vi "06a-arrays.vi"() -> ()   [LabVIEW 2018, in "LV-0mq-Julia_roundtrip-lib.lvlib"]
uses:
  LV-0mq-Julia_roundtrip-lib.lvlib
  Server or client state.ctl
  detailed error info.ctl
  StackFrame.ctl
  Commands.ctl
  72a46192-383e-4ee5-9465-71670922b82a.vi
  ef5408d4-6538-41d1-b296-fda05a71e4b0.vi
  d2cb43a9-9305-42fb-ad58-bce983510195.vi
  e4efb182-1b04-4d49-96a3-1defebd055ea.vi
  ebebf057-8b7e-42d1-8726-0ed76f361650.vi
  72a46192-383e-4ee5-9465-71670922b82a.vi/ea2ca31c-a649-493c-8d06-3a8000b732b1.vi
  ef5408d4-6538-41d1-b296-fda05a71e4b0.vi/365813fc-9c19-4b31-a490-477dd90e6dd4.vi
  d2cb43a9-9305-42fb-ad58-bce983510195.vi/e28c4e1c-617d-4a26-8291-f58a5accd33d.vi
  d2cb43a9-9305-42fb-ad58-bce983510195.vi/697b26af-9cff-4296-98ec-fa9d12ca8fdc.vi
  d2cb43a9-9305-42fb-ad58-bce983510195.vi/17159f77-75f5-4b7b-8d47-844af2eb1bcd.vi
  e4efb182-1b04-4d49-96a3-1defebd055ea.vi/c831fe72-f3ce-4847-96da-e1889b23ddae.vi
  e4efb182-1b04-4d49-96a3-1defebd055ea.vi/ef51326b-c369-4f95-bb54-a6ec3719e99a.vi
  ebebf057-8b7e-42d1-8726-0ed76f361650.vi/2896c3ac-7382-471b-957d-23d54ee9f1a8.vi
  ebebf057-8b7e-42d1-8726-0ed76f361650.vi/710b0f88-80e8-4b85-a109-d5d9dfaa7844.vi
  72a46192-383e-4ee5-9465-71670922b82a.vi/ea2ca31c-a649-493c-8d06-3a8000b732b1.vi/4cda02a8-52b1-4797-9517-7736628fdc16.vi
  ef5408d4-6538-41d1-b296-fda05a71e4b0.vi/365813fc-9c19-4b31-a490-477dd90e6dd4.vi/c1bf83d8-4e50-4008-8373-782bae7d23a9.vi
  e4efb182-1b04-4d49-96a3-1defebd055ea.vi/c831fe72-f3ce-4847-96da-e1889b23ddae.vi/9c4cdaea-65f9-4c6c-8a66-2fd1ac6f4f5c.vi
  e4efb182-1b04-4d49-96a3-1defebd055ea.vi/c831fe72-f3ce-4847-96da-e1889b23ddae.vi/3acea7b0-1723-4660-a8ee-e10d34bc4f15.vi
  ebebf057-8b7e-42d1-8726-0ed76f361650.vi/2896c3ac-7382-471b-957d-23d54ee9f1a8.vi/1bedb906-9d55-4714-9acf-3a7596d20d1c.vi
  ebebf057-8b7e-42d1-8726-0ed76f361650.vi/2896c3ac-7382-471b-957d-23d54ee9f1a8.vi/27a3c6cf-df38-46c5-966e-0597bcc583ab.vi
  72a46192-383e-4ee5-9465-71670922b82a.vi/ea2ca31c-a649-493c-8d06-3a8000b732b1.vi/4cda02a8-52b1-4797-9517-7736628fdc16.vi/f6bd3a2a-1504-4020-af9c-daf7937f7973.vi
  ef5408d4-6538-41d1-b296-fda05a71e4b0.vi/365813fc-9c19-4b31-a490-477dd90e6dd4.vi/c1bf83d8-4e50-4008-8373-782bae7d23a9.vi/fa26639b-d519-4ace-9d6a-dd3a988d1d0b.vi
  e4efb182-1b04-4d49-96a3-1defebd055ea.vi/c831fe72-f3ce-4847-96da-e1889b23ddae.vi/9c4cdaea-65f9-4c6c-8a66-2fd1ac6f4f5c.vi/fa7cffbf-0952-4399-bf7e-4cf3444aec21.vi
  ebebf057-8b7e-42d1-8726-0ed76f361650.vi/2896c3ac-7382-471b-957d-23d54ee9f1a8.vi/1bedb906-9d55-4714-9acf-3a7596d20d1c.vi/32202c8e-48ac-4eff-9f06-aea6b9e0f0c2.vi
  jl-scripts path.vi
  check ID validity.vi
  bindata_descr to JSON.vi
  check cluster field names.vi
  concat JSON.vi
  <vilib>/Utility/error.llb/Error Cluster From Error Code.vi
panel:
  out "inverted matrix":dbl[][](array[numeric])=[[1.0, 0.0, 5.0], [4.0, 2.0, 1.0], [2.0, 2.0, 3.0]] format="%#.4g"
  out "determinant":dbl
  out "Solution Vector":dbl[](array[numeric]) format="%.2f"
  in  "Known Vector":dbl[](array[numeric])=[22.0, 14.0, 18.0]
  in  "Input Matrix":dbl[][](array[numeric])=[[1.0, 0.0, 5.0], [4.0, 2.0, 1.0], [2.0, 2.0, 3.0]]
  in  "next":bool
  out "detailed error info":T1
  out "current error":errorcluster
  out "final error":errorcluster
  out "short err code":u8
  in  "stop":bool
  out "ZMQ timeout":bool
  out "Julia script file path":path
  out "temporary script path":path
  out "Jl Server state":T3
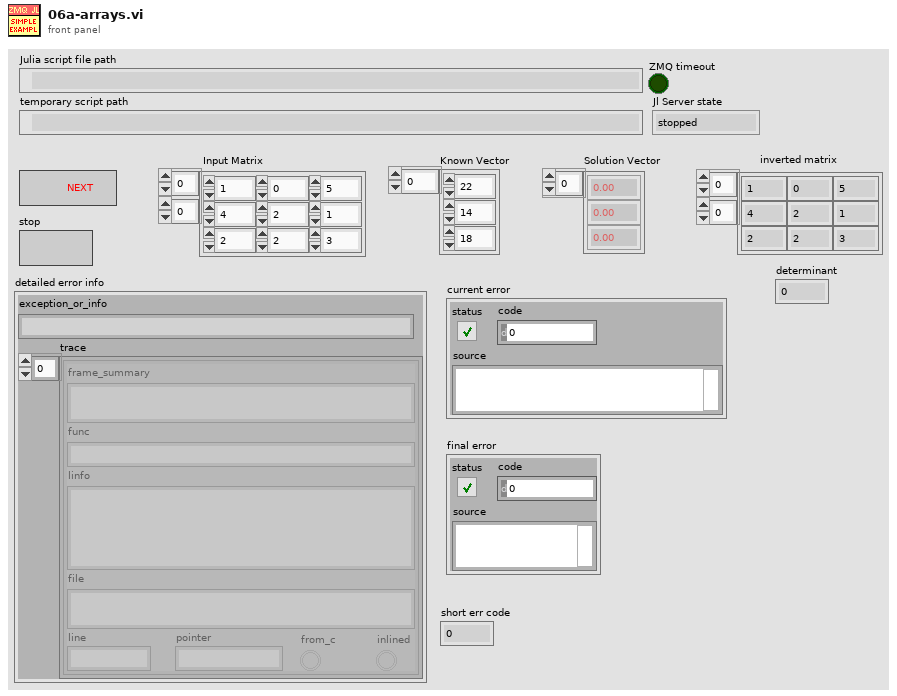
[diagram p1: front panel]
types:
  T1 = typedef "LV-0mq-Julia_roundtrip-lib.lvlib/detailed error info.ctl" = cluster{"exception_or_info":string, "trace":T2[]}
  T2 = typedef "LV-0mq-Julia_roundtrip-lib.lvlib/StackFrame.ctl" = cluster{"frame_summary":string, "func":string, "linfo":string, "file":string, "line":i32, "pointer":u64, "from_c":bool, "inlined":bool}
  T3 = typedef "LV-0mq-Julia_roundtrip-lib.lvlib/Server or client state.ctl" = enum16{"stopped", "running", "unknown"}
  T4 = typedef "LV-0mq-Julia_roundtrip-lib.lvlib/Commands.ctl" = enum16{"Start Jl-server & Init LV-client", "Send request & Get response ", "Stop Jl-server & Cleanup LV-client", "Cleanup LV-client", "Start Jl-server", "Stop Jl-server", "Init LV-Client", "Cleanup LV-Client", "(not allowed)", "Set LV Client state", "Set Jl Server state", "set ZMQ timeout", "read ZMQ timeout", "read-out state"}
  T5 = typedef "LV-0mq-Julia_roundtrip-lib.lvlib/Bindata&description.ctl" = cluster{"bindata_descr":T6[], "bindata":u8[]}
  T6 = typedef "LV-0mq-Julia_roundtrip-lib.lvlib/Bindata description.ctl" = cluster{"nofbytes":i32, "numtype":string, "start":i32, "arrdims":i32[], "kwarg_name":string, "category":string}
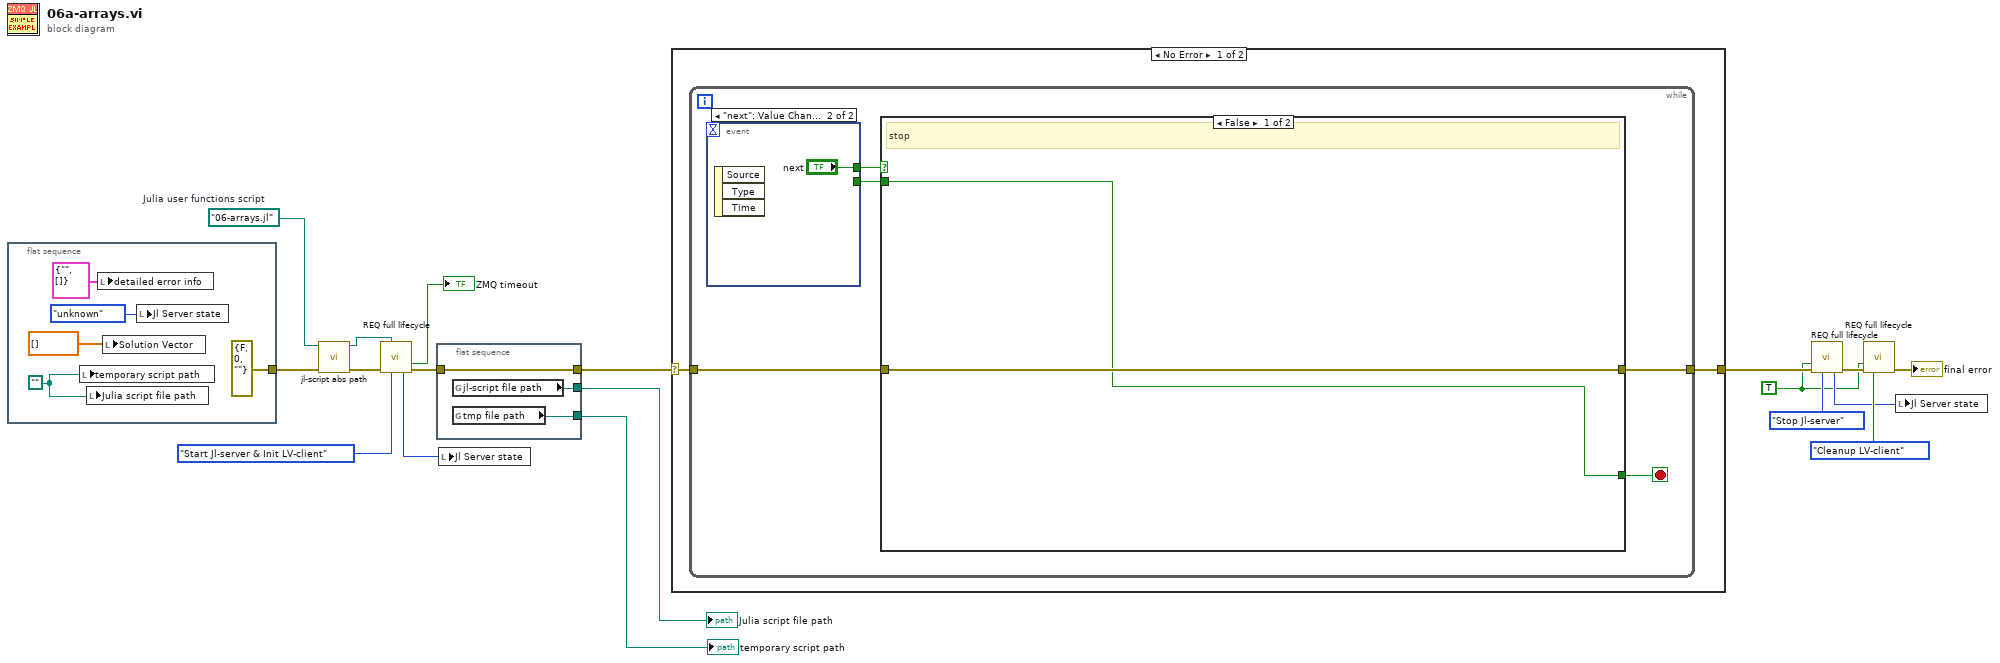
[diagram p0: block diagram]
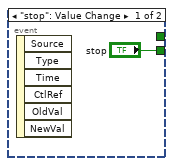
[diagram p2: hidden frame]
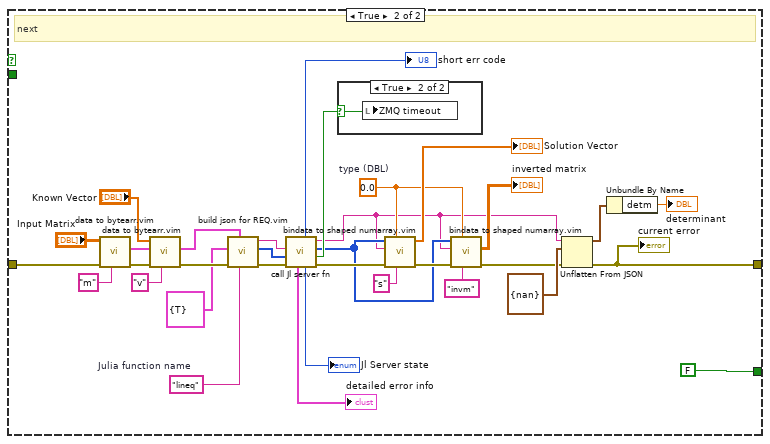
[diagram p3: hidden frame]
diagram:
  w4 = path "06-arrays.jl"  # Julia user functions script
  w1 = TRUE ("Force command")
  n1 = flat-sequence {
    tunnel: [errorcluster {"status"=FALSE, "code"=0, "source"=""} ("error in (no error)")] -> w2
    frame #0 {
      w19 = path ""
      n2 = local write "temporary script path"(w19) -> ()
      n3 = local write "Julia script file path"(w19) -> ()
      n4 = local write "detailed error info"(T1 {"exception_or_info"="", "trace"=[]} ("detailed error info")) -> ()
      n5 = local write "Solution Vector"(dbl[] [] ("Server response")) -> ()
      n6 = local write "Jl Server state"(Server_or_client_state."unknown" ("Jl Server state out")) -> ()
    }
  }
  n7 = call "jl-script abs path.vi"("error in (no error)"=w2, "Julia user functions script"=w4) -> ("error out"=w5:errorcluster, "script abs path"=w6:path)  [unwired: 8 in]
  n8 = call "REQ full lifecycle.vi"("Julia user functions script"=w6, "error in"=w5, "command"=Commands."Start Jl-server & Init LV-client") -> ("timeout?"=→"ZMQ timeout":bool, "Jl Server state out"=w8:T3, "error out"=w7:errorcluster)  [unwired: 6 in, 4 out]
  n9 = flat-sequence {
    tunnel: [w26] -> w13
    tunnel: w7 -> [w26]
    tunnel: [w25] -> w11
    tunnel: [w24] -> w12
    frame #0 {
      n10 = global read "jl-scripts path.vi" "jl-script file path"() -> (w25:path)
      n11 = global read "jl-scripts path.vi" "tmp file path"() -> (w24:path)
    }
  }
  n12 = local write "Jl Server state"(w8) -> ()
  n13 = case shown="No Error" w13 {
    selector: w13 -> [w27 w72]
    tunnel: [w28 w72] -> w18
    frame No Error {
      n14 = while {
        tunnel: w27 -> [w32]
        tunnel: [w33] -> w28
        stop <- w30 stop-if-true
        n15 = event shown="[1] \"next\": Value Change" {
          selector: _ -> [_ _]
          dyn-events: _ -> [_ _]
          timeout: _ -> [_ _]
          tunnel: [_ "next"] -> w31
          tunnel: ["stop" _] -> w29
          event "stop": Value Change {
            n16 = event-data() -> ()  [unwired: 1 in, 6 out]
          }
          event "next": Value Change {
            n17 = event-data() -> ()  [unwired: 1 in, 3 out]
          }
        }
        n18 = case shown="False" w31 {
          tunnel: [w37 w46] -> w33
          tunnel: w32 -> [w37 w56]
          tunnel: [w36 FALSE ("stop this VI only")] -> w30
          tunnel: w29 -> [w36 _]
          frame False {
            # "stop"
          }
          frame True {
            w40 = 0.0  # type (DBL)
            w62 = "lineq"  # Julia function name
            # "next"
            n19 = call "data to bytearr.vim"("kwarg_name"="m", "error in (no error)"=w56, "data in"="Input Matrix") -> ("error out"=w60:errorcluster, "Bindata & descr out"=w59:T5)  [unwired: 6 in, 1 out]
            n20 = call "data to bytearr.vim"("kwarg_name"="v", "error in (no error)"=w60, "Bindata & descr in"=w59, "data in"="Known Vector") -> ("error out"=w57:errorcluster, "Bindata & descr out"=w53:T5)  [unwired: 5 in, 1 out]
            n21 = call "build json for REQ.vim"("fun2call"=w62, "Bindata & descr in"=w53, "error in (no error)"=w57, "Arguments 2"=cluster{"invert":bool} {"invert"=TRUE}) -> ("error out"=w67:errorcluster, "bindata out"=w68:u8[], "JSON string out"=w69:string)  [unwired: 5 in]
            n22 = call "call Jl server fn.vi"("error in (no error)"=w67, "binary data in"=w68, "JSON string in"=w69) -> ("error out"=w52:errorcluster, "timeout?"=w63:bool, "binary data received"=w42:u8[], "JSON received"=w38:string, "Jl Server state out"=→"Jl Server state":T3, "return code"=→"short err code":u8, "detailed error info"=→"detailed error info":T1)  [unwired: 2 in]
            n23 = case shown="True" w63 {
              selector: w63 -> [_ w71]
              frame False {
              }
              frame True {
                n24 = local write "ZMQ timeout"(w71) -> ()
              }
            }
            n25 = call "bindata to shaped numarray.vim"("kwarg_name"="s", "data type"=w40, "error in (no error)"=w52, "bindata_descr"=w38, "binary data"=w42) -> ("error out"=w44:errorcluster, "numarray 1D"=→"Solution Vector":dbl[])  [unwired: 3 in, 2 out]
            n26 = call "bindata to shaped numarray.vim"("kwarg_name"="invm", "data type"=w40, "error in (no error)"=w44, "bindata_descr"=w38, "binary data"=w42) -> ("error out"=w43:errorcluster, "numarray 2D"=→"inverted matrix":dbl[][])  [unwired: 3 in, 2 out]
            n27 = Unflatten From JSON(JSON string=w38, type and defaults=cluster{"detm":dbl} {"detm"=nan}, error in (no error)=w43) -> (value=w47:cluster{"detm":dbl}, error out=w46:errorcluster)  [unwired: 4 in]
            "current error" <- w46
            n28 = Unbundle By Name(w47) -> ("detm"=→"determinant":dbl)
          }
        }
      }
    }
    frame Error {
    }
  }
  n29 = call "REQ full lifecycle.vi"("Force command"=w1, "error in"=w18, "command"=Commands."Stop Jl-server") -> ("Jl Server state out"=w10:T3, "error out"=w16:errorcluster)  [unwired: 6 in, 5 out]
  n30 = call "REQ full lifecycle.vi"("Force command"=w1, "error in"=w16, "command"=Commands."Cleanup LV-client") -> ("error out"=→"final error":errorcluster)  [unwired: 6 in, 6 out]
  n31 = local write "Jl Server state"(w10) -> ()
  "temporary script path" <- w12
  "Julia script file path" <- w11
